vi "TEST To String Set Key.vi"() -> ()   [LabVIEW 2013, in "Carya Config.lvclass"]
doc: "Copyright 2018, Carya Automatisering, Wiebe Walstra."
uses:
  Carya Config.lvclass
panel:
  out "String 3":string
  out "String":string
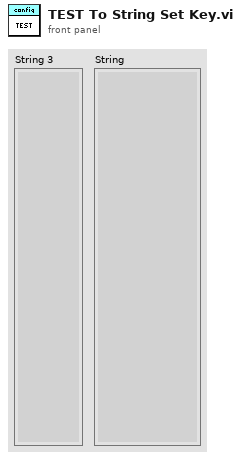
[diagram p1: front panel]
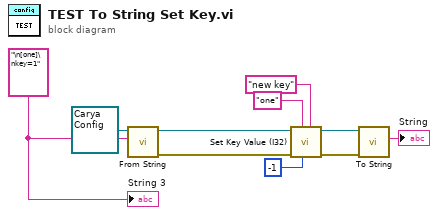
[diagram p0: block diagram]
diagram:
  w9 = "\n[one]\nkey=1" ("String")
  n1 = call-dynamic "From String.vi"("String"=w9, "Carya Config in"=refnum<class "Carya Config.lvclass"> refnum) -> ("error out"=w7:errorcluster, "Carya Config out"=w6:refnum<class "Carya Config.lvclass">)  [unwired: 7 in, 1 out]
  n2 = call "Set Key Value (I32).vi"("Key name"="new key", "Key value"=-1, "Section name"="one", "error in (no error)"=w7, "Carya Config in"=w6) -> ("error out"=w4:errorcluster, "Carya Config out"=w5:refnum<class "Carya Config.lvclass">)  [unwired: 2 in, 3 out]
  n3 = call-dynamic "To String.vi"("error in (no error)"=w4, "Carya Config in"=w5) -> ("String"=→"String":string)  [unwired: 7 in, 2 out]
  "String 3" <- w9
